vi "CODMn通讯.vi"() -> ()   [LabVIEW 2016, in "斯坦道CODMn.lvlib"]
uses:
  <vilib>/Plasmionique/MB Master/MB_Master_TCP/MB_Master_TCP.lvclass
  D:/Program Files (x86)/National Instruments/LabVIEW 2016/vi.lib/Plasmionique/MB Master/MB_Master/MB_Master.lvclass
  <vilib>/Plasmionique/MB Master/MB Master.lvlib
  <vilib>/Utility/config.llb/NI_LVConfig.lvlib
  <vilib>/Plasmionique/MB Master/MB_Master/MB_Master.lvclass
panel:
  in  "读取数据":bool
  in  "释放串口":bool
  in  "打开串口":bool
  out "队列中元素数量":i32
  out "元素":cluster{"命令":string}[](array[cluster])
  out "待处理插入数量":i32
  out "读取公式":u16[](array[numeric])
  out "读取参数":u16[](array[numeric])
  out "数据存储":u16[](array[numeric])
  out "温度":bool[](array[boolean])
  out "M输出点":bool[](array[boolean])
  out "ORP、时间":u16[](array[numeric])
  out "测量状态":u16[](array[numeric])
  out "通讯状态":bool
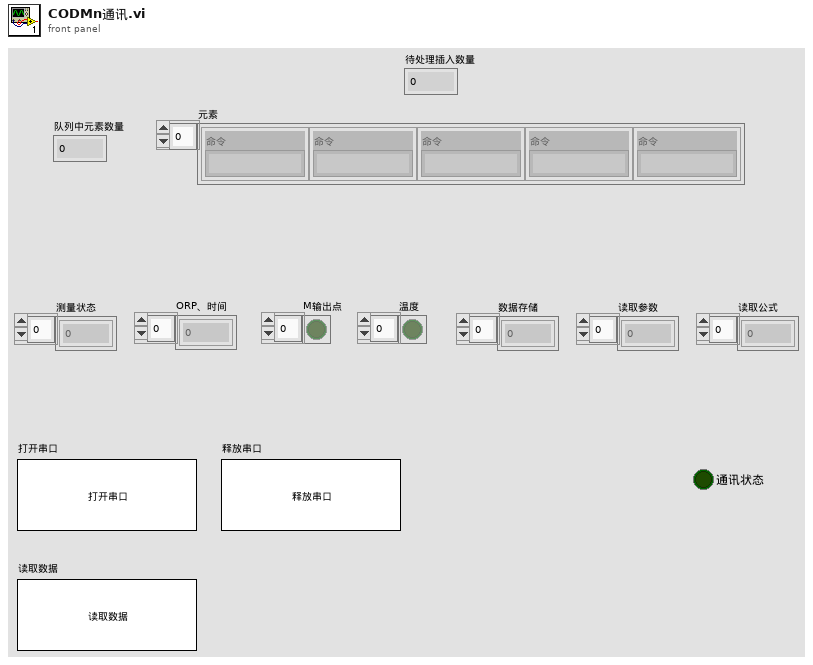
[diagram p1: front panel]
types:
  T1 = typedef "NI_LVConfig.lvlib/Config Data RefNum.ctl" = refnum<k1>
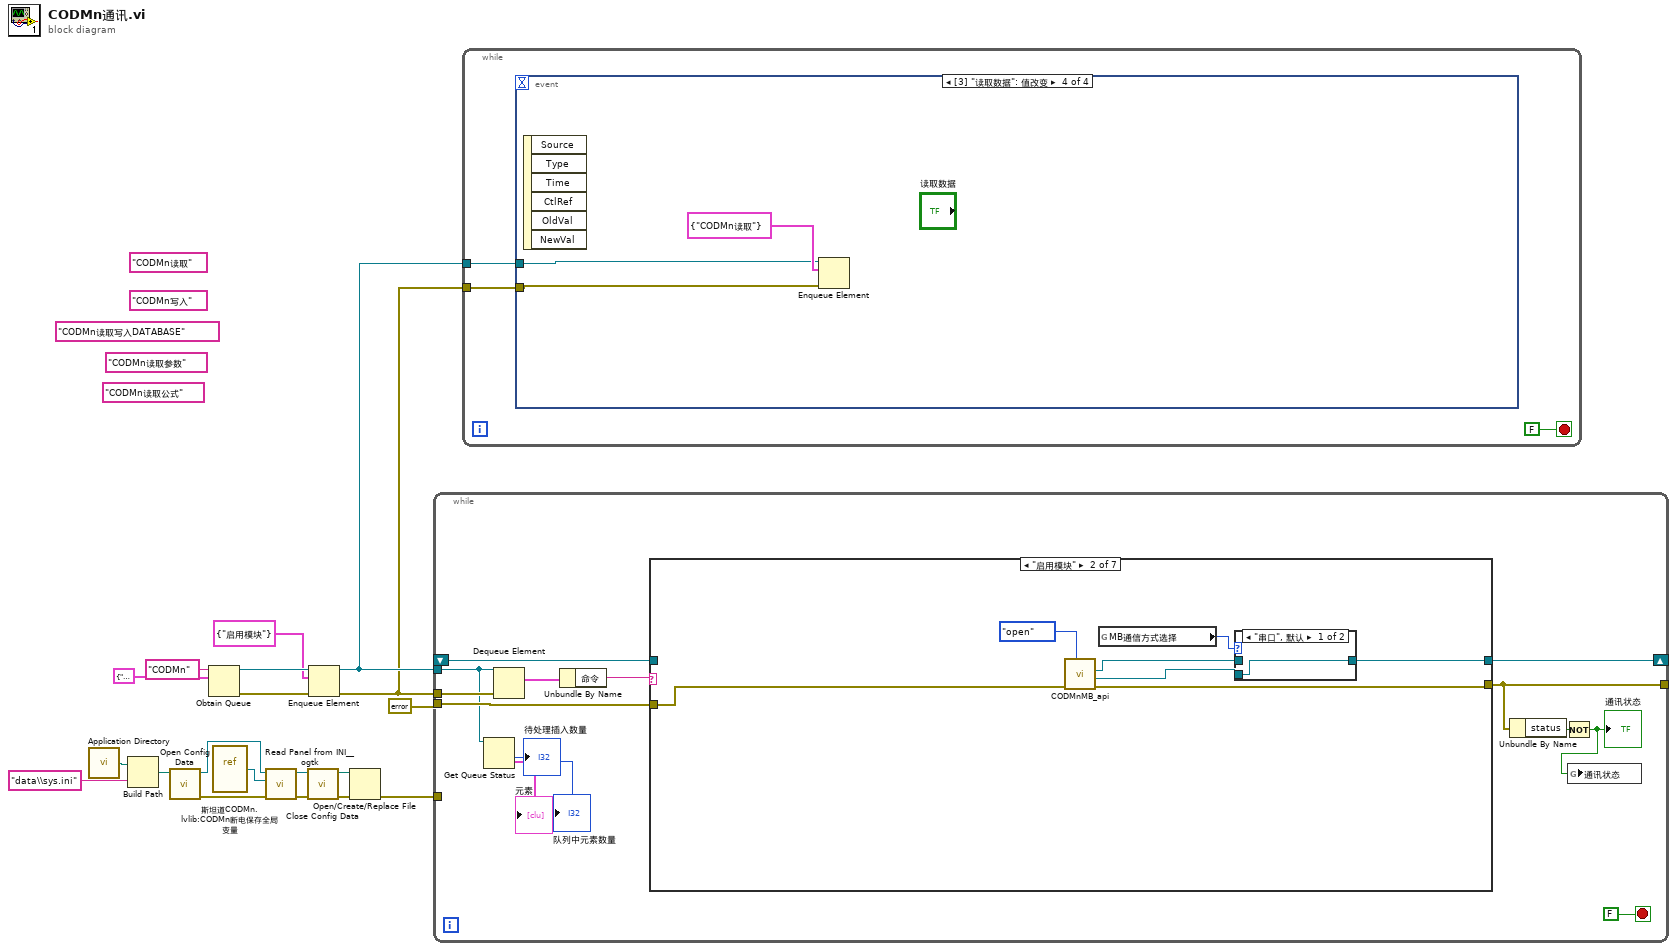
[diagram p0: block diagram]
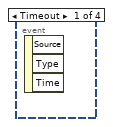
[diagram p2: hidden frame]
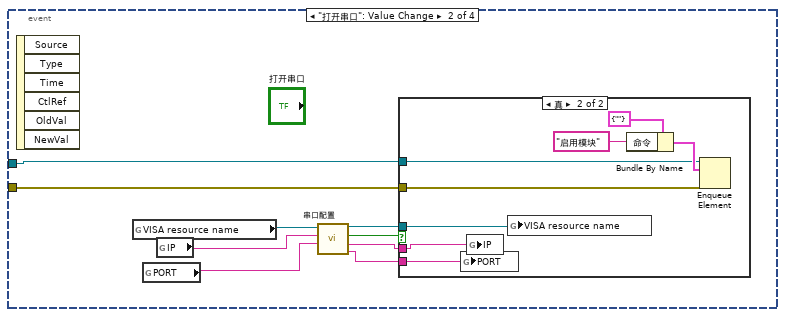
[diagram p3: hidden frame]
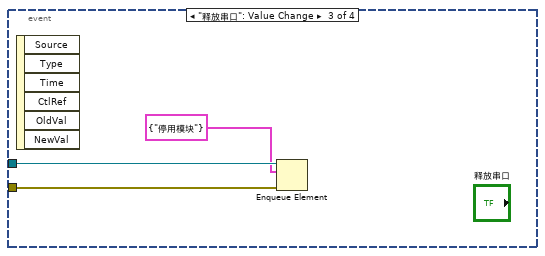
[diagram p5: hidden frame]
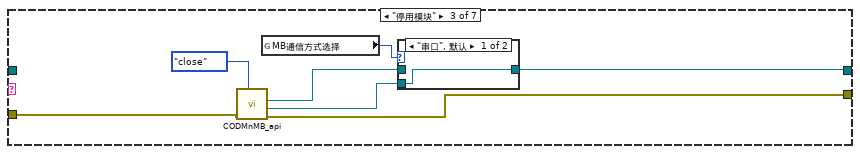
[diagram p8: hidden frame]
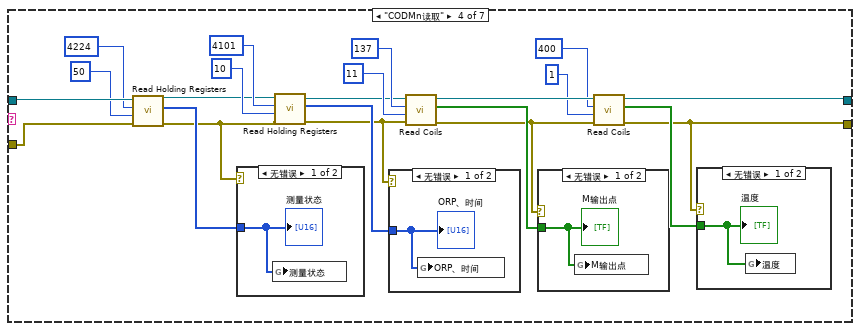
[diagram p10: hidden frame]
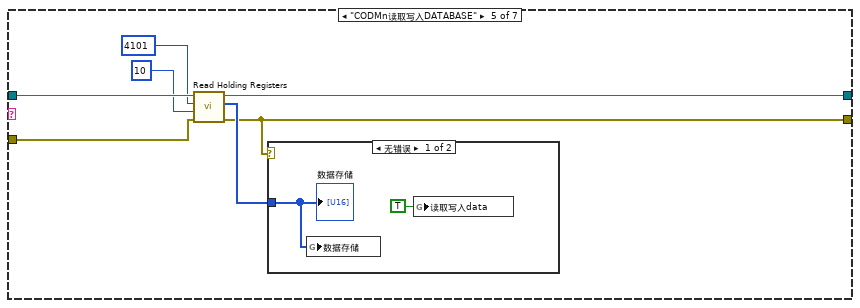
[diagram p15: hidden frame]
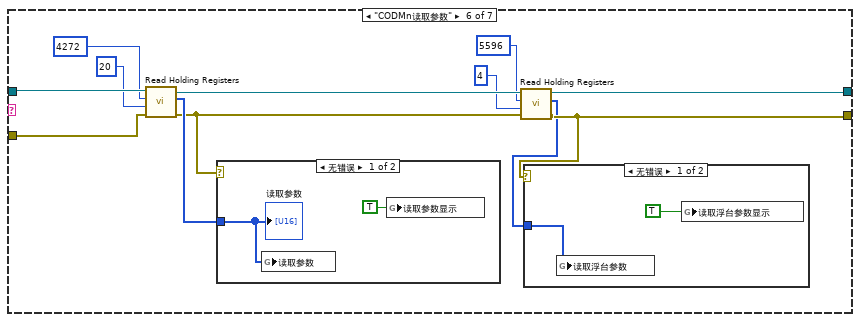
[diagram p17: hidden frame]
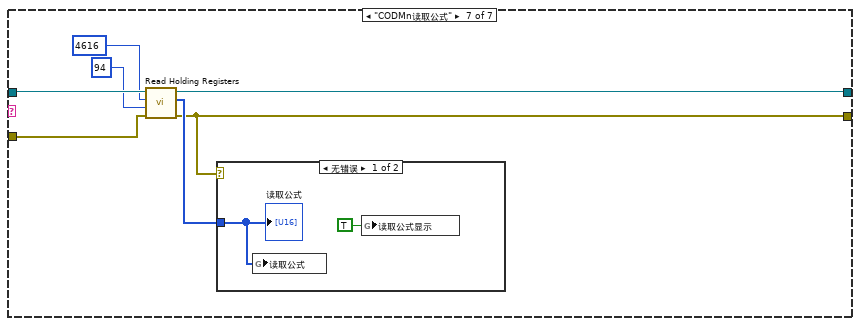
[diagram p20: hidden frame]
diagram:
  (unwired) "CODMn读取公式" ("名称（未命名）")
  (unwired) "CODMn读取写入DATABASE" ("名称（未命名）")
  (unwired) "CODMn读取参数" ("名称（未命名）")
  (unwired) "CODMn读取" ("名称（未命名）")
  (unwired) "CODMn写入" ("名称（未命名）")
  n1 = call <vilib>:"Application Directory.vi"() -> ("Application Directory"=w13:path)
  n2 = Build Path(base path=w13, name or relative path="data\\sys.ini" ("名称或相对路径")) -> (appended path=w11:path)
  n3 = call <vilib>:"Open Config Data.vi"("configuration file path"=w11) -> ("error out"=w7:errorcluster, "refnum"=w10:T1)  [unwired: 8 in, 1 out]
  n4 = Obtain Queue(name (unnamed)="CODMn" ("名称（未命名）"), element data type=cluster{"命令":string} {"命令"="启用模块"} ("元素")) -> (queue out=w16:refnum<queue>, error out=w15:errorcluster)  [unwired: 3 in, 1 out]
  n5 = vi-ref "斯坦道CODMn.lvlib:CODMn断电保存全局变量.vi"() -> (w9:refnum<vi>)
  n6 = call <userlib>:"Read Panel from INI__ogtk.vi"("error in (no error)"=w7, "VI ref"=w9, "refnum"=w10) -> ("error out"=w6:errorcluster, "refnum out"=w8:T1)  [unwired: 7 in]
  n7 = call <vilib>:"Close Config Data.vi"("error in (no error)"=w6, "refnum"=w8) -> ("error out"=w5:errorcluster, "file path"=w4:path)  [unwired: 8 in]
  n8 = Enqueue Element(queue=w16, element=cluster{"命令":string} {"命令"="启用模块"} ("元素"), error in (no error)=w15) -> (queue out=w2:refnum<queue>, error out=w1:errorcluster)  [unwired: 1 in, 1 out]
  n9 = Open/Create/Replace File(file path (use dialog)=w4, error in=w5) -> (error out=w3:errorcluster)  [unwired: 4 in, 2 out]
  n10 = while {
    tunnel: w2 -> [w23]
    tunnel: w1 -> [w32]
    tunnel: [w24] -> _
    shift-right: [w28] -> _
    shift-left: _ -> [w27]
    tunnel: errorcluster {"status"=FALSE, "code"=0, "source"=""} ("error out") -> [w26]
    tunnel: w3 -> [_]
    stop <- FALSE stop-if-true
    n11 = Get Queue Status(queue=w23) -> (# pending insert=→"待处理插入数量":i32, # elements in queue=→"队列中元素数量":i32, elements=→"元素":cluster{"命令":string}[])  [unwired: 2 in, 5 out]
    n12 = Dequeue Element(queue=w23, error in (no error)=w32) -> (element=w31:cluster{"命令":string})  [unwired: 1 in, 3 out]
    n13 = Unbundle By Name(w31) -> ("命令"=w30:string)
    n14 = case shown="\"启用模块\"" w30 {
      tunnel: [w35 w36 w46 w61 w82 w91 w108] -> w28
      tunnel: [w34 w42 w49 w54 w80 w90 w107] -> w24
      tunnel: w27 -> [w35 _ _ w75 w86 w100 w111]
      tunnel: w26 -> [w34 w40 w50 w74 w83 w99 w110]
      frame Default {
      }
      frame "启用模块" {
        n15 = call "CODMnMB_api.vi"("STEP"=enum16{"open", "read", "write", "close"}."open", "Error in"=w40) -> ("error out"=w42:errorcluster, "MB session out"=w37:refnum<class "MB_Master.lvclass">, "MB_TCP session"=w38:refnum<class "MB_Master_TCP.lvclass">)  [unwired: 6 in, 1 out]
        n16 = global read "CODMn断电保存全局变量.vi" "MB通信方式选择"() -> (w39:enum16{"串口", "TCP"})
        n17 = case shown="\"串口\", 默认" w39 {
          tunnel: w38 -> [_ w44]
          tunnel: w37 -> [w43 _]
          tunnel: [w43 w44] -> w36
          frame "串口", Default {
          }
          frame "TCP" {
          }
        }
      }
      frame "停用模块" {
        n18 = call "CODMnMB_api.vi"("STEP"=enum16{"open", "read", "write", "close"}."close", "Error in"=w50) -> ("error out"=w49:errorcluster, "MB session out"=w47:refnum<class "MB_Master.lvclass">, "MB_TCP session"=w45:refnum<class "MB_Master_TCP.lvclass">)  [unwired: 6 in, 1 out]
        n19 = global read "CODMn断电保存全局变量.vi" "MB通信方式选择"() -> (w48:enum16{"串口", "TCP"})
        n20 = case shown="\"串口\", 默认" w48 {
          tunnel: w45 -> [_ w53]
          tunnel: w47 -> [w52 _]
          tunnel: [w52 w53] -> w46
          frame "串口", Default {
          }
          frame "TCP" {
          }
        }
      }
      frame "CODMn读取" {
        n21 = call <vilib>:"Read Holding Registers.vi"("error in (no error)"=w74, "quantity"=u16 50 ("number of holding registers"), "starting address"=u16 4224, "MB session in"=w75) -> ("error out"=w65:errorcluster, "Registers"=w71:u16[], "MB session out"=w66:refnum<class "MB_Master.lvclass">)  [unwired: 5 in]
        n22 = case shown="无错误" w65 {
          tunnel: w71 -> [w79 _]
          frame No Error {
            n23 = global write "COD读取DATA全局.vi" "测量状态"(w79) -> ()
            "测量状态" <- w79
          }
          frame Error {
          }
        }
        n24 = call <vilib>:"Read Holding Registers.vi"("error in (no error)"=w65, "quantity"=u16 10, "starting address"=u16 4101, "MB session in"=w66) -> ("error out"=w60:errorcluster, "Registers"=w64:u16[], "MB session out"=w63:refnum<class "MB_Master.lvclass">)  [unwired: 5 in]
        n25 = case shown="无错误" w60 {
          tunnel: w64 -> [w78 _]
          frame No Error {
            n26 = global write "COD读取DATA全局.vi" "ORP、时间"(w78) -> ()
            "ORP、时间" <- w78
          }
          frame Error {
          }
        }
        n27 = call <vilib>:"Read Coils.vi"("error in (no error)"=w60, "quantity"=u16 11, "starting address"=u16 137, "MB session in"=w63) -> ("error out"=w58:errorcluster, "Coils"=w59:bool[], "MB session out"=w62:refnum<class "MB_Master.lvclass">)  [unwired: 5 in]
        n28 = case shown="无错误" w58 {
          tunnel: w59 -> [w77 _]
          frame No Error {
            n29 = global write "COD读取DATA全局.vi" "M输出点"(w77) -> ()
            "M输出点" <- w77
          }
          frame Error {
          }
        }
        n30 = call <vilib>:"Read Coils.vi"("error in (no error)"=w58, "quantity"=u16 1, "starting address"=u16 400, "MB session in"=w62) -> ("error out"=w54:errorcluster, "Coils"=w55:bool[], "MB session out"=w61:refnum<class "MB_Master.lvclass">)  [unwired: 5 in]
        n31 = case shown="无错误" w54 {
          tunnel: w55 -> [w76 _]
          frame No Error {
            n32 = global write "COD读取DATA全局.vi" "温度"(w76) -> ()
            "温度" <- w76
          }
          frame Error {
          }
        }
      }
      frame "CODMn读取写入DATABASE" {
        n33 = call <vilib>:"Read Holding Registers.vi"("error in (no error)"=w83, "quantity"=u16 10 ("number of holding registers"), "starting address"=u16 4101, "MB session in"=w86) -> ("error out"=w80:errorcluster, "Registers"=w81:u16[], "MB session out"=w82:refnum<class "MB_Master.lvclass">)  [unwired: 5 in]
        n34 = case shown="无错误" w80 {
          tunnel: w81 -> [w88 _]
          frame No Error {
            n35 = global write "COD读取DATA全局.vi" "数据存储"(w88) -> ()
            n36 = global write "COD读取DATA全局.vi" "读取写入data"(TRUE ("读取参数显示")) -> ()
            "数据存储" <- w88
          }
          frame Error {
          }
        }
      }
      frame "CODMn读取参数" {
        n37 = call <vilib>:"Read Holding Registers.vi"("error in (no error)"=w99, "quantity"=u16 20 ("number of holding registers"), "starting address"=u16 4272, "MB session in"=w100) -> ("error out"=w94:errorcluster, "Registers"=w96:u16[], "MB session out"=w95:refnum<class "MB_Master.lvclass">)  [unwired: 5 in]
        n38 = case shown="无错误" w94 {
          tunnel: w96 -> [w104 _]
          frame No Error {
            n39 = global write "COD读取DATA全局.vi" "读取参数"(w104) -> ()
            n40 = global write "COD读取DATA全局.vi" "读取参数显示"(TRUE ("读取参数显示")) -> ()
            "读取参数" <- w104
          }
          frame Error {
          }
        }
        n41 = call <vilib>:"Read Holding Registers.vi"("error in (no error)"=w94, "quantity"=u16 4, "starting address"=u16 5596, "MB session in"=w95) -> ("error out"=w90:errorcluster, "Registers"=w89:u16[], "MB session out"=w91:refnum<class "MB_Master.lvclass">)  [unwired: 5 in]
        n42 = case shown="无错误" w90 {
          tunnel: w89 -> [w102 _]
          frame No Error {
            n43 = global write "COD读取DATA全局.vi" "读取浮台参数"(w102) -> ()
            n44 = global write "COD读取DATA全局.vi" "读取浮台参数显示"(TRUE ("读取参数显示")) -> ()
          }
          frame Error {
          }
        }
      }
      frame "CODMn读取公式" {
        n45 = call <vilib>:"Read Holding Registers.vi"("error in (no error)"=w110, "quantity"=u16 94 ("number of holding registers"), "starting address"=u16 4616, "MB session in"=w111) -> ("error out"=w107:errorcluster, "Registers"=w109:u16[], "MB session out"=w108:refnum<class "MB_Master.lvclass">)  [unwired: 5 in]
        n46 = case shown="无错误" w107 {
          tunnel: w109 -> [w113 _]
          frame No Error {
            n47 = global write "COD读取DATA全局.vi" "读取公式"(w113) -> ()
            n48 = global write "COD读取DATA全局.vi" "读取公式显示"(TRUE ("读取参数显示")) -> ()
            "读取公式" <- w113
          }
          frame Error {
          }
        }
      }
    }
    n49 = Unbundle By Name(w24) -> ("status"=w29:bool)
    n50 = Not(x=w29) -> (.not. x?=w25:bool)
    "通讯状态" <- w25
    n51 = global write "COD读取DATA全局.vi" "通讯状态"(w25) -> ()
  }
  n52 = while {
    tunnel: w2 -> [w115]
    tunnel: w1 -> [w114]
    stop <- FALSE stop-if-true
    n53 = event shown="[3] \"读取数据\": 值改变" {
      selector: _ -> [_ _ _ _]
      dyn-events: _ -> [_ _ _ _]
      timeout: _ -> [_ _ _ _]
      tunnel: w115 -> [_ w122 w136 w138]
      tunnel: w114 -> [_ w121 w135 w137]
      event Timeout {
        n54 = event-data() -> ()  [unwired: 1 in, 3 out]
      }
      event "打开串口": Value Change {
        n55 = event-data() -> ()  [unwired: 1 in, 6 out]
        n56 = global read "CODMn断电保存全局变量.vi" "VISA resource name"() -> (w125:refnum<visa-resource-name>)
        n57 = global read "CODMn断电保存全局变量.vi" "PORT"() -> (w119:string)
        n58 = global read "CODMn断电保存全局变量.vi" "IP"() -> (w120:string)
        n59 = call "串口配置.vi"("PORT"=w119, "IP"=w120, "请选择串口:"=w125) -> ("PORT 2"=w117:string, "IP 2"=w118:string, "确认 2"=w123:bool, "VISA资源名称 2"=w124:refnum<visa-resource-name>)  [unwired: 5 in]
        n60 = case shown="真" w123 {
          tunnel: w124 -> [_ w133]
          tunnel: w122 -> [_ w129]
          tunnel: w121 -> [_ w128]
          tunnel: w118 -> [_ w127]
          tunnel: w117 -> [_ w126]
          frame False {
          }
          frame True {
            n61 = global write "CODMn断电保存全局变量.vi" "PORT"(w126) -> ()
            n62 = global write "CODMn断电保存全局变量.vi" "IP"(w127) -> ()
            n63 = global write "CODMn断电保存全局变量.vi" "VISA resource name"(w133) -> ()
            n64 = Bundle By Name(cluster=cluster{"命令":string} {"命令"=""} ("元素"), "命令"="启用模块" ("名称（未命名）")) -> (w130:cluster{"命令":string})
            n65 = Enqueue Element(queue=w129, element=w130, error in (no error)=w128) -> ()  [unwired: 1 in, 3 out]
          }
        }
      }
      event "释放串口": Value Change {
        n66 = event-data() -> ()  [unwired: 1 in, 6 out]
        n67 = Enqueue Element(queue=w136, element=cluster{"命令":string} {"命令"="停用模块"} ("元素"), error in (no error)=w135) -> ()  [unwired: 1 in, 3 out]
      }
      event "读取数据": Value Change {
        n68 = event-data() -> ()  [unwired: 1 in, 6 out]
        n69 = Enqueue Element(queue=w138, element=cluster{"命令":string} {"命令"="CODMn读取"} ("元素"), error in (no error)=w137) -> ()  [unwired: 1 in, 3 out]
      }
    }
  }
